vi "Format string with manual word wrap .vi"(5 "Chars per line":i8, 6 "String":string) -> (2 "String with manual Word Wrap":string)   [LabVIEW 2009]
doc: "Takes a string and automatically word-wraps it based on the Chars per line input. VI will search for a space after it reaches the specified number of characters and append a carriage return to the line.\n\nIf \"Chars per line\" is -1 it word-wrapping is disabled."
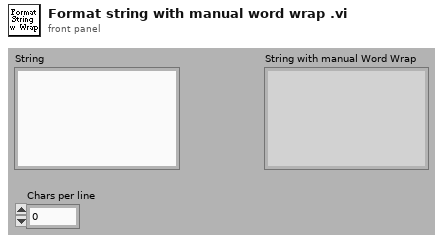
[diagram p1: front panel]
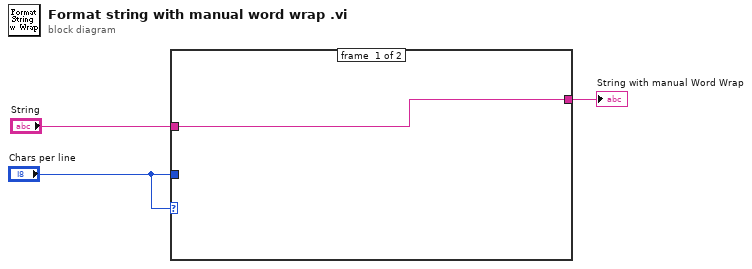
[diagram p0: block diagram]
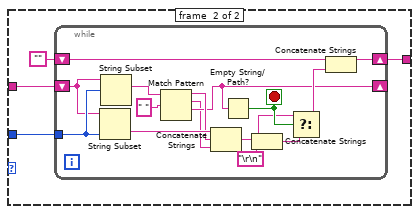
[diagram p2: hidden frame]
diagram:
  n1 = case shown="Default" "Chars per line" {
    tunnel: [w4 w8] -> w3
    tunnel: "Chars per line" -> [_ w7]
    tunnel: "String" -> [w4 w6]
    frame #0 {
    }
    frame #1 {
      n2 = while {
        tunnel: w7 -> [w20]
        shift-right: [w21] -> w8
        shift-left: "" -> [w22]
        shift-right: [w10] -> _
        shift-left: w6 -> [w19]
        stop <- w18 stop-if-true
        n3 = String Subset(string=w19, length (rest)=w20) -> (substring=w13:string)  [unwired: 1 out]
        n4 = String Subset(string=w19, offset (0)=w20) -> (substring=w11:string)  [unwired: 1 out]
        n5 = Match Pattern(string=w11, regular expression=" ") -> (before substring=w12:string, match substring=w9:string, after substring=w10:string)  [unwired: 2 out]
        n6 = Concatenate Strings(w13, w12, w9) -> (w14:string)
        n7 = Empty String/Path?(string/path=w10) -> (empty?=w18:bool)
        n8 = Concatenate Strings(w14, "\r\n") -> (w17:string)
        n9 = Select(t=w14, s=w18, f=w17) -> (s? t:f=w16:string)
        n10 = Concatenate Strings(w22, w16) -> (w21:string)
      }
    }
  }
  "String with manual Word Wrap" <- w3
